vi "Lockin.DAQ.Configure Sweep 3.vi"(8 "error in (no error)":errorcluster, 11 "Lockin.DAQ in":refnum<class "Lockin.DAQ.lvclass">) -> (0 "error out":errorcluster, 3 "Lockin.DAQ out":refnum<class "Lockin.DAQ.lvclass">)   [LabVIEW 2016, in "Lockin.DAQ.lvclass"]
uses:
  Lockin.DAQ.lvclass
  Lockin.DAQ.lvclass/Lockin.DAQ.ctl
  Typedefs/Function-enum.ctl
panel:
  out "Frequency (Hz)":dbl
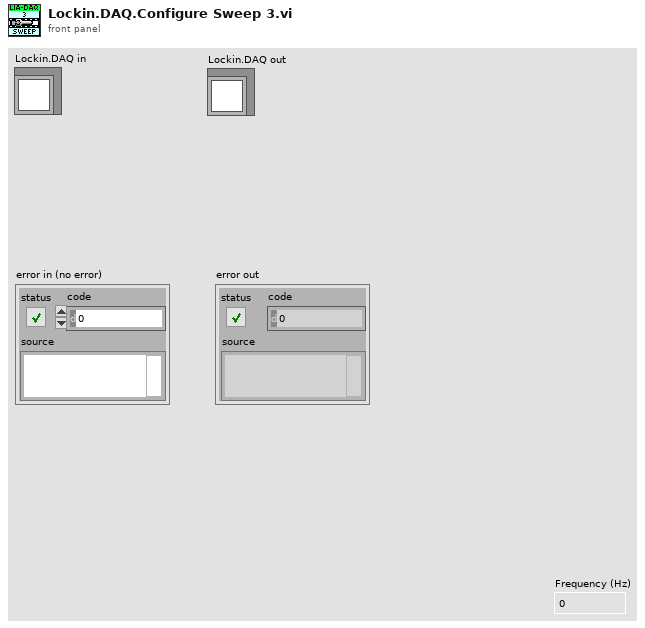
[diagram p1: front panel]
types:
  T1 = typedef "Lockin.DAQ.lvclass/AO-cluster.ctl" = cluster{"Ch":i32[], "Amp (V)":dbl[], "DC (V)":dbl[], "f (Hz)":dbl[], "Phase (°)":dbl[], "Function":T2[], "Sweep?":bool[]}
  T2 = typedef "Lockin.DAQ.lvclass/Function-enum.ctl" = enum16{"Sine", "Triangle", "Square", "Sawtooth"}
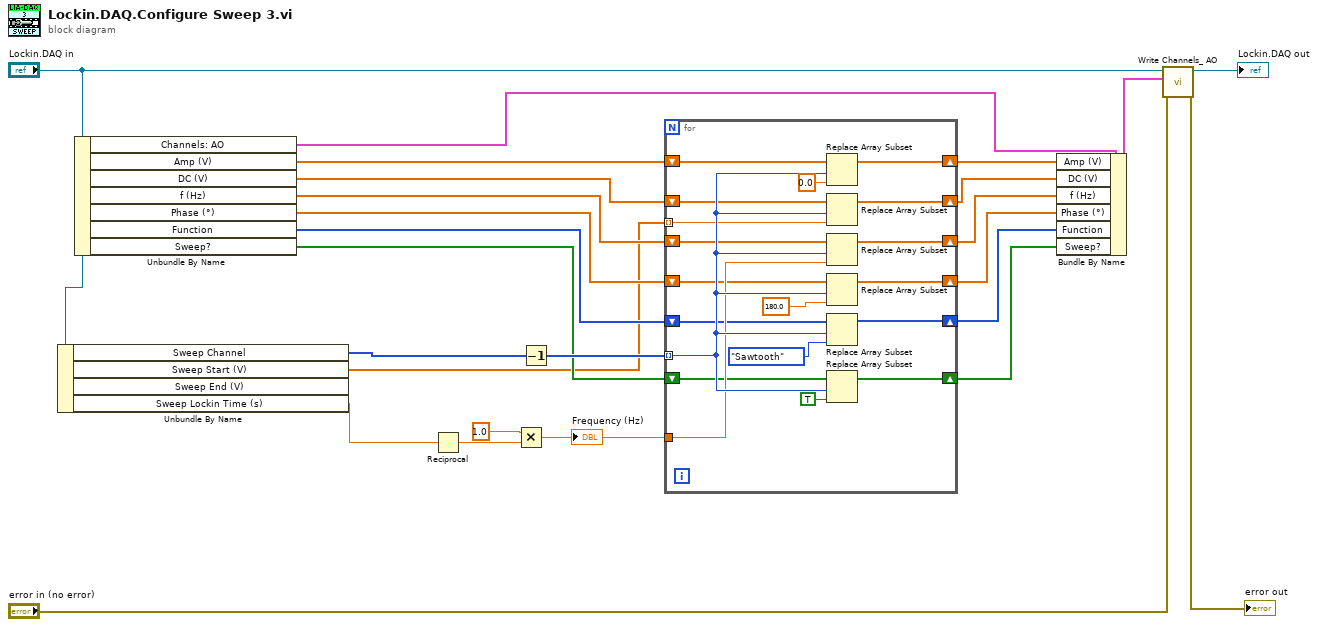
[diagram p0: block diagram]
diagram:
  n1 = Unbundle By Name("Lockin.DAQ in") -> ("Sweep Channel"=w6:i32[], "Sweep Start (V)"=w3:dbl[], "Sweep Lockin Time (s)"=w4:dbl)  [unwired: 1 out]
  n2 = Unbundle By Name("Lockin.DAQ in") -> ("Channels: AO"=w2:T1, "Amp (V)"=w17:dbl[], "DC (V)"=w16:dbl[], "f (Hz)"=w15:dbl[], "Phase (°)"=w14:dbl[], "Function"=w13:T2[], "Sweep?"=w12:bool[])
  n3 = Reciprocal(x=w4) -> (1/x=w21:dbl)
  n4 = Multiply(x=1.0, y=w21) -> (x*y=w19:dbl)
  "Frequency (Hz)" <- w19
  n5 = Decrement(x=w6) -> (x-1=w20:i32[])
  n6 = for {
    tunnel: w20 -> [w41] mode=indexing
    tunnel: w19 -> [w40]
    tunnel: w3 -> [w26] mode=indexing
    shift-right: [w33] -> w1
    shift-left: w17 -> [w39]
    shift-right: [w32] -> w11
    shift-left: w16 -> [w38]
    shift-right: [w31] -> w10
    shift-left: w15 -> [w37]
    shift-right: [w30] -> w9
    shift-left: w14 -> [w36]
    shift-right: [w29] -> w8
    shift-left: w13 -> [w35]
    shift-right: [w28] -> w7
    shift-left: w12 -> [w34]
    n7 = Replace Array Subset(array=w39, new element=0.0 ("new element/subarray"), index=w41) -> (w33:dbl[])
    n8 = Replace Array Subset(array=w38, new element=w26, index=w41) -> (w32:dbl[])
    n9 = Replace Array Subset(array=w37, new element=w40, index=w41) -> (w31:dbl[])
    n10 = Replace Array Subset(array=w36, new element=180.0 ("new element/subarray"), index=w41) -> (w30:dbl[])
    n11 = Replace Array Subset(array=w35, new element=Function-enum."Sawtooth" ("new element/subarray"), index=w41) -> (w29:T2[])
    n12 = Replace Array Subset(array=w34, new element=TRUE ("new element/subarray"), index=w41) -> (w28:bool[])
  }
  n13 = Bundle By Name(cluster=w2, "Amp (V)"=w1, "DC (V)"=w11, "f (Hz)"=w10, "Phase (°)"=w9, "Function"=w8, "Sweep?"=w7) -> (w22:T1)
  n14 = call "Write Channels_ AO.vi"("error in (no error)"="error in (no error)", "Channels: AO"=w22, "Lockin.DAQ"="Lockin.DAQ in") -> ("error out"=→"error out":errorcluster, "Lockin.DAQ out"=→"Lockin.DAQ out":refnum<class "Lockin.DAQ.lvclass">)  [unwired: 7 in]
